vi "Test_TripTime.vi"(2 "error in (no error)":errorcluster, 3 "Break in":bool[](array[boolean]), 4 "Time":i32, 5 "Trip Time in":i32[](array[numeric])) -> (0 "error out":errorcluster, 1 "Trip Time out":i32[](array[numeric]))   [LabVIEW 2015]
doc: "firstTripped?：首次脱扣状态，0：从未脱扣，1：已经脱扣\nBreak：断路器的状态，0：脱扣，1：未脱扣\nTrippedTime：脱扣时间\npreTrippedTime：之前的脱扣时间"
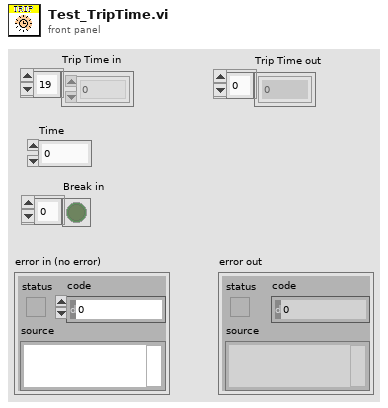
[diagram p1: front panel]
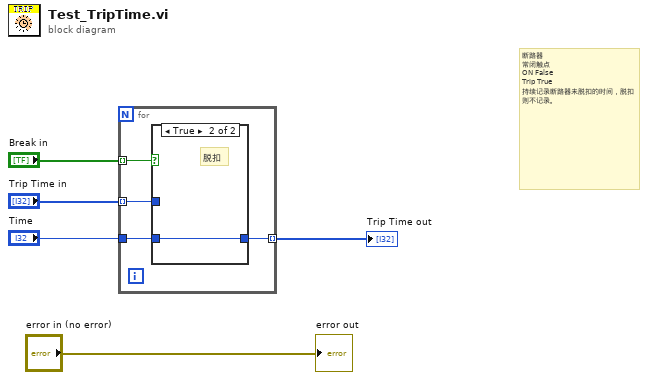
[diagram p0: block diagram]
diagram:
  # "断路器\n常闭触点\nON False\nTrip True\n持续记录断路器未脱扣的时间，脱扣则不记录。"
  n1 = for {
    tunnel: "Break in" -> [w9] mode=indexing
    tunnel: "Time" -> [w8]
    tunnel: [w7] -> w4 mode=indexing
    tunnel: "Trip Time in" -> [w6] mode=indexing
    n2 = case shown="True" w9 {
      tunnel: [w10 w11] -> w7
      tunnel: w8 -> [_ w11]
      tunnel: w6 -> [w10 _]
      frame False {
      }
      frame True {
        # "脱扣"
      }
    }
  }
  "Trip Time out" <- w4
  "error out" <- "error in (no error)"
